vi "SwerveDriveLogic.vi"(9 "Speeds":dbl[](array[numeric]), 10 "AngleSetpoints":dbl[](array[numeric]), 11 "AngleEncoders":dbl[](array[numeric])) -> (2 "AngleMotorsReversed":bool[](array[boolean]), 3 "AngleMotorOutputs":dbl[](array[numeric]))   [LabVIEW 2018]
uses:
  <vilib>/Rock Robotics/Network Tables/NT Write Numeric Array.vi
  <vilib>/addons/control/pid/pid.llb/PID (DBL).vi
  <vilib>/Rock Robotics/Network Tables/NT Write Boolean Array.vi
  <vilib>/addons/control/pid/NI_PID_pid.lvlib
panel:
  out "Back right module":dbl(knob)
  out "Back left module":dbl(knob)
  out "Front left module":dbl(knob)
  out "Front right module":dbl(knob)
  in  "PID gains":T1={"proportional gain (Kc)"=0.02, "integral time (Ti, min)"=0.0, "derivative time (Td, min)"=0.0} {"derivative time (Td, min)" format="%.15f"; "integral time (Ti, min)" format="%.3f"; "proportional gain (Kc)" format="%.3f"}
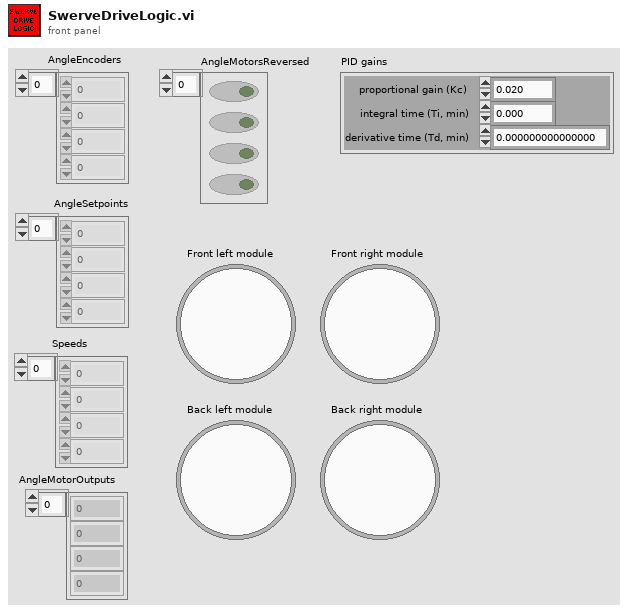
[diagram p1: front panel]
types:
  T1 = cluster{"proportional gain (Kc)":dbl, "integral time (Ti, min)":dbl, "derivative time (Td, min)":dbl}
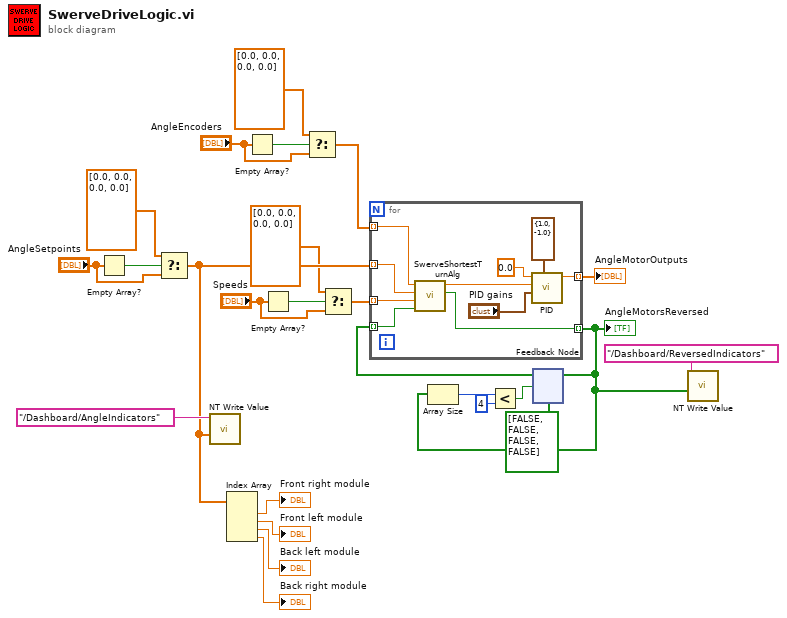
[diagram p0: block diagram]
diagram:
  n1 = Empty Array?(array="AngleSetpoints") -> (empty?=w15:bool)
  n2 = Select(t=dbl[] [0.0, 0.0, 0.0, 0.0] ("AngleSetpoints"), s=w15, f="AngleSetpoints") -> (s? t:f=w14:dbl[])
  n3 = call-poly <vilib>:"NT Write Value.vi"("Numeric Array"=w14, "Name"="/Dashboard/AngleIndicators") -> ()  [unwired: 9 in, 1 out]
  n4 = Index Array(array=w14) -> (element #1=→"Front right module":dbl, element #2=→"Front left module":dbl, element #3=→"Back left module":dbl, element #4=→"Back right module":dbl)  [unwired: 4 in]
  n5 = Empty Array?(array="AngleEncoders") -> (empty?=w18:bool)
  n6 = Empty Array?(array="Speeds") -> (empty?=w12:bool)
  n7 = Select(t=dbl[] [0.0, 0.0, 0.0, 0.0] ("AngleSetpoints"), s=w18, f="AngleEncoders") -> (s? t:f=w7:dbl[])
  n8 = Select(t=dbl[] [0.0, 0.0, 0.0, 0.0] ("AngleSetpoints"), s=w12, f="Speeds") -> (s? t:f=w10:dbl[])
  n9 = feedback #1(bool[] [FALSE, FALSE, FALSE, FALSE]) -> (w3:bool[])
  n10 = for {
    tunnel: w3 -> [w30] mode=indexing
    tunnel: w14 -> [w32] mode=indexing
    tunnel: [w34] -> w25 mode=indexing
    tunnel: [w26] -> w2 mode=indexing
    tunnel: w7 -> [w29] mode=indexing
    tunnel: w10 -> [w28] mode=indexing
    n11 = call "SwerveShortestTurnAlg.vi"("SwerveMotorsFlipped?"=w30, "SwerveSpeed"=w28, "AngleSetpoint"=w32, "AngleEncoder"=w29) -> ("FlipSwerveMotors"=w26:bool, "PIDInput"=w27:dbl)  [unwired: 6 in]
    n12 = call-poly <vilib>:"PID.vi"("output range"=cluster{"output high":dbl, "output low":dbl} {"output high"=1.0, "output low"=-1.0}, "PID gains"="PID gains", "process variable"=w27, "setpoint"=0.0) -> ("output"=w34:dbl)  [unwired: 6 in, 1 out]
  }
  "AngleMotorsReversed" <- w2
  "AngleMotorOutputs" <- w25
  n13 = Array Size(array=w2) -> (size(s)=w4:i32)
  n14 = Less?(x=w4, y=4) -> (x < y?=w5:bool)
  n15 = feedback-in #1(w2, w5) -> ()
  n16 = call-poly <vilib>:"NT Write Value.vi"("Boolean Array"=w2, "Name"="/Dashboard/ReversedIndicators") -> ()  [unwired: 9 in, 1 out]
